vi "helper_upload.vi"(4 "chunk_size_bytes":i64=157286400, 6 "timeout_ms":i32=10000, 8 "error in (no error)":errorcluster, 9 "file":string, 10 "path":string, 11 "filepath":path) -> (0 "error out":errorcluster, 3 "filepath":string)   [LabVIEW 2015, in "lv-dropbox.lvlib" / "v2.lvlib"]
uses:
  v2.lvlib
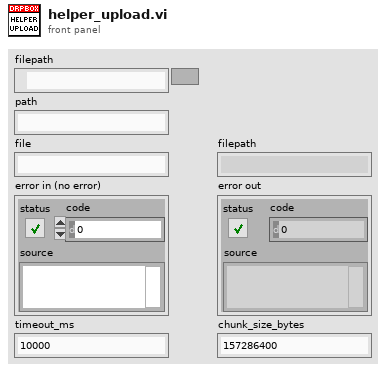
[diagram p1: front panel]
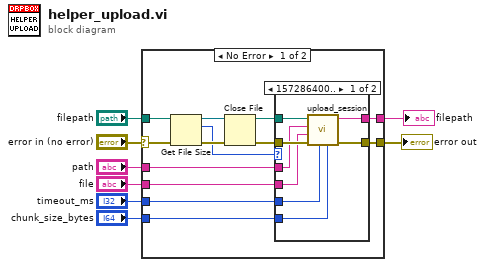
[diagram p0: block diagram]
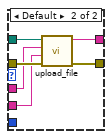
[diagram p2: hidden frame]
diagram:
  n1 = case shown="No Error" "error in (no error)" {
    selector: "error in (no error)" -> [w21 w36]
    tunnel: "filepath" -> [w18 _]
    tunnel: "path" -> [w15 _]
    tunnel: "file" -> [w14 _]
    tunnel: [w13 w36] -> w4
    tunnel: "timeout_ms" -> [w12 _]
    tunnel: "chunk_size_bytes" -> [w11 _]
    tunnel: [w10 _] -> w1
    frame No Error {
      n2 = Get File Size(file=w18, error in=w21) -> (refnum out=w20:refnum<file>, size (in bytes)=w9:i64, 0:w19:errorcluster)
      n3 = Close File(refnum=w20, error in=w19) -> (path=w16:path, error out=w17:errorcluster)
      n4 = case shown="157286400.." w9 {
        tunnel: w17 -> [w28 w34]
        tunnel: w16 -> [w29 w35]
        tunnel: w15 -> [w27 w33]
        tunnel: w14 -> [w26 w32]
        tunnel: [w25 w31] -> w13
        tunnel: w12 -> [w24 _]
        tunnel: w11 -> [w23 _]
        tunnel: [w22 w30] -> w10
        frame 157286400.. {
          n5 = call "upload_session.vi"("chunk_size_bytes"=w23, "timeout_ms"=w24, "error in (no error)"=w28, "file"=w26, "path"=w27, "filepath"=w29) -> ("error out"=w25:errorcluster, "filepath"=w22:string)  [unwired: 4 in]
        }
        frame Default {
          n6 = call "upload_file.vi"("error in (no error)"=w34, "file"=w32, "path"=w33, "filepath"=w35) -> ("error out"=w31:errorcluster, "filepath"=w30:string)  [unwired: 6 in]
        }
      }
    }
    frame Error {
    }
  }
  "error out" <- w4
  "filepath" <- w1
